vi "Stepper motor-Example.vi"() -> ()   [LabVIEW 2013]
uses:
  <vilib>/LabVIEW Interface for Arduino/Type Defs/Connection Type.ctl
  <vilib>/LabVIEW Interface for Arduino/Type Defs/Board Type.ctl
  <vilib>/LabVIEW Interface for Arduino/LabVIEW Interface for Arduino.lvlib
panel:
  in  "?":bool
  in  "RPM Control":dbl(knob) scale=0.0..6.0
  in  "Continuious Mode":bool
  in  "Half Step":bool
  in  "CW":bool
  # "Control Panel"
  # "CCW"
  # "Full Step"
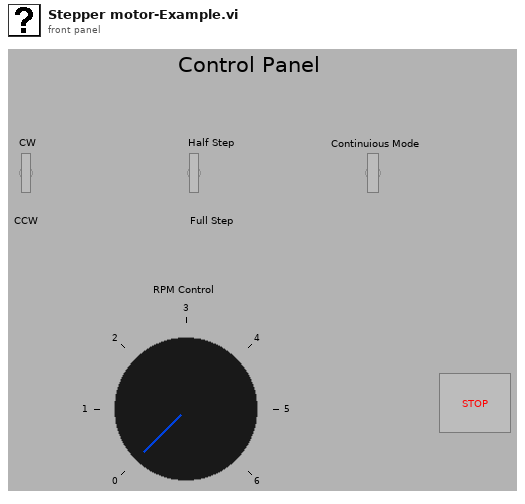
[diagram p1: front panel]
types:
  T1 = typedef "LabVIEW Interface for Arduino.lvlib/Board Type.ctl" = enum16{"Uno", "Dimuelanove w/Atmega 328", "Mega 2560"}
  T2 = typedef "LabVIEW Interface for Arduino.lvlib/Connection Type.ctl" = enum8{"USB / Serial", "XBEE", "BlueSmirf (Bluetooth)"}
  T3 = typedef "LabVIEW Interface for Arduino.lvlib/Arduino Resource.ctl" = cluster{"VISA resource":refnum<visa-resource-name>, "Board Type":T1, "Connection Type":enum8{"USB / Serial"}, "Bytes Per Packet (15)":u8}
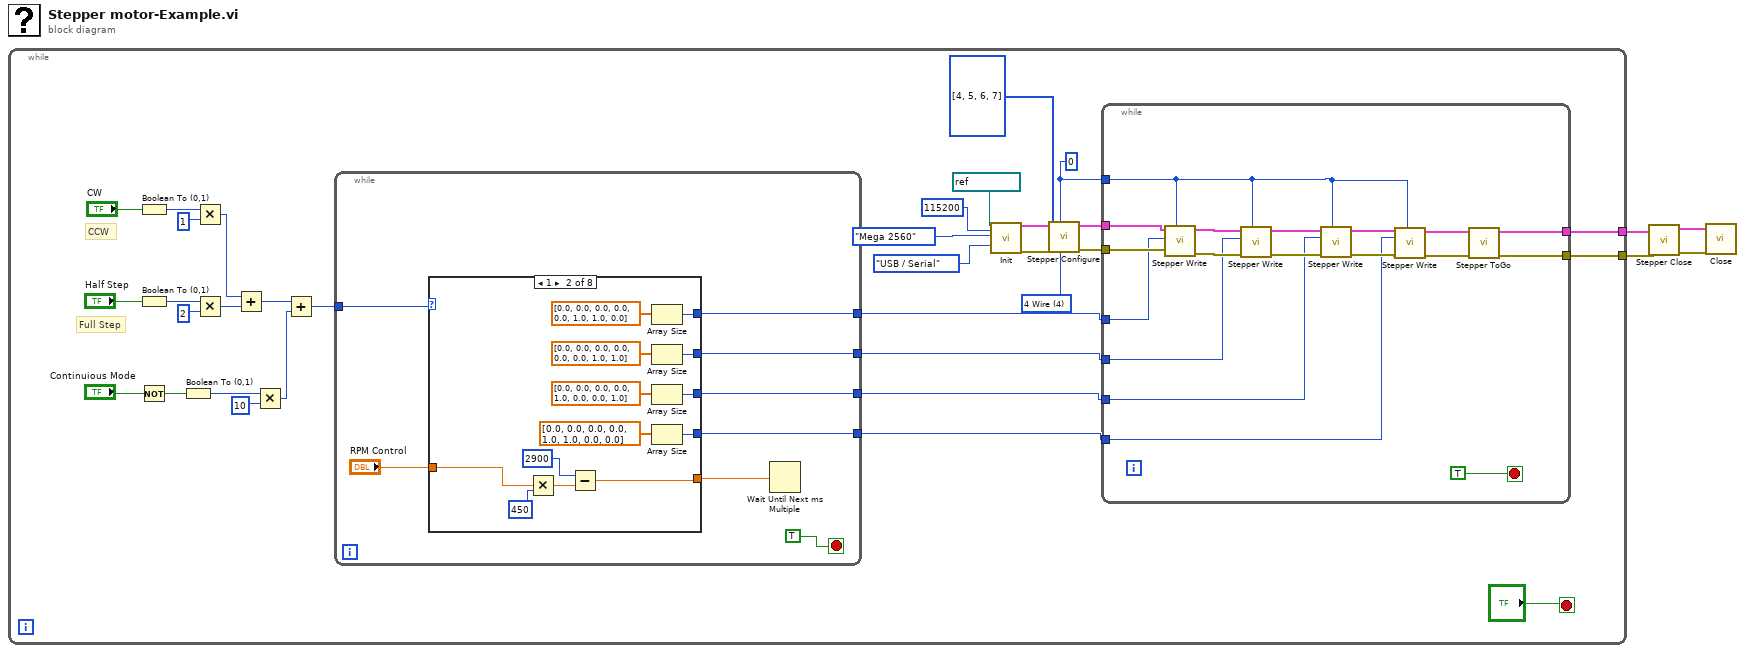
[diagram p0: block diagram]
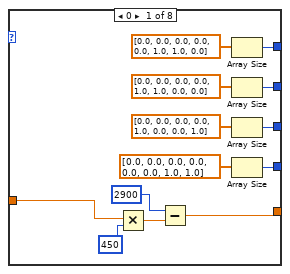
[diagram p2: hidden frame]
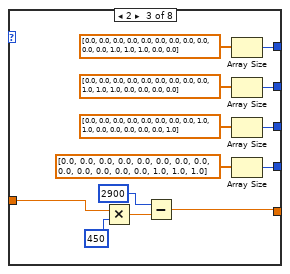
[diagram p3: hidden frame]
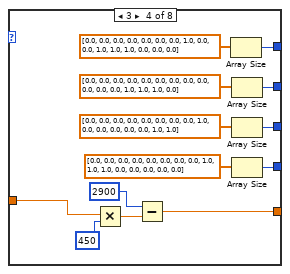
[diagram p4: hidden frame]
diagram:
  n1 = while {
    tunnel: [w6] -> w4
    tunnel: [w5] -> w3
    stop <- "?" stop-if-true
    w17 = u8 4 items=["2 Wire (Pulse & Direction)"=1, "2 Wire"=2, "4 Wire"=4, "EasyDriver"=6, "AF Motor Shield (Stepper 1 & 2 Only)"=5] ("Control Method")
    w21 = u8 0 ("Stepper #")
    # "Full Step"
    # "CCW"
    n2 = Boolean To (0,1)(Boolean="CW") -> (0, 1=w37:i16)
    n3 = Boolean To (0,1)(Boolean="Half Step") -> (0, 1=w34:i16)
    n4 = Not(x="Continuious Mode") -> (.not. x?=w31:bool)
    n5 = Boolean To (0,1)(Boolean=w31) -> (0, 1=w29:i16)
    n6 = Multiply(x=w37, y=1) -> (x*y=w30:i32)
    n7 = Multiply(x=w34, y=2) -> (x*y=w25:i32)
    n8 = Add(x=w30, y=w25) -> (x+y=w27:i32)
    n9 = Multiply(x=w29, y=10) -> (x*y=w26:i32)
    n10 = Add(x=w27, y=w26) -> (x+y=w23:i32)
    n11 = while {
      tunnel: w23 -> [w61]
      tunnel: [w59] -> w11
      tunnel: [w58] -> w10
      tunnel: [w57] -> w9
      tunnel: [w56] -> w8
      stop <- TRUE stop-if-true
      n12 = case "CW Full" shown="1" w61 {
        tunnel: [w72 w85 w98 w111 _ _ _ _] -> w56
        tunnel: [w71 w84 w97 w110 _ _ _ _] -> w58
        tunnel: [w70 w83 w96 w109 _ _ _ _] -> w57
        tunnel: [w69 w82 w95 w108 _ _ _ _] -> w59
        tunnel: "RPM Control" -> [w65 w78 w91 w103 _ _ _ _]
        tunnel: [w64 w77 w90 w106 _ _ _ _] -> w62
        frame 0 {
          n13 = Multiply(x=w65, y=450) -> (x*y=w67:dbl)
          n14 = Subtract(x=2900, y=w67) -> (x-y=w64:dbl)
          n15 = Array Size(array=dbl[] [0.0, 0.0, 0.0, 0.0, 0.0, 1.0, 1.0, 0.0]) -> (size(s)=w69:i32)
          n16 = Array Size(array=dbl[] [0.0, 0.0, 0.0, 0.0, 1.0, 1.0, 0.0, 0.0]) -> (size(s)=w71:i32)
          n17 = Array Size(array=dbl[] [0.0, 0.0, 0.0, 0.0, 1.0, 0.0, 0.0, 1.0]) -> (size(s)=w70:i32)
          n18 = Array Size(array=dbl[] [0.0, 0.0, 0.0, 0.0, 0.0, 0.0, 1.0, 1.0]) -> (size(s)=w72:i32)
        }
        frame 1 {
          n19 = Multiply(x=w78, y=450) -> (x*y=w80:dbl)
          n20 = Subtract(x=2900, y=w80) -> (x-y=w77:dbl)
          n21 = Array Size(array=dbl[] [0.0, 0.0, 0.0, 0.0, 0.0, 1.0, 1.0, 0.0]) -> (size(s)=w82:i32)
          n22 = Array Size(array=dbl[] [0.0, 0.0, 0.0, 0.0, 0.0, 0.0, 1.0, 1.0]) -> (size(s)=w84:i32)
          n23 = Array Size(array=dbl[] [0.0, 0.0, 0.0, 0.0, 1.0, 0.0, 0.0, 1.0]) -> (size(s)=w83:i32)
          n24 = Array Size(array=dbl[] [0.0, 0.0, 0.0, 0.0, 1.0, 1.0, 0.0, 0.0]) -> (size(s)=w85:i32)
        }
        frame 2 {
          n25 = Multiply(x=w91, y=450) -> (x*y=w93:dbl)
          n26 = Subtract(x=2900, y=w93) -> (x-y=w90:dbl)
          n27 = Array Size(array=dbl[] [0.0, 0.0, 0.0, 0.0, 0.0, 0.0, 0.0, 0.0, 0.0, 0.0, 0.0, 1.0, 1.0, 1.0, 0.0, 0.0]) -> (size(s)=w95:i32)
          n28 = Array Size(array=dbl[] [0.0, 0.0, 0.0, 0.0, 0.0, 0.0, 0.0, 0.0, 0.0, 1.0, 1.0, 1.0, 0.0, 0.0, 0.0, 0.0]) -> (size(s)=w97:i32)
          n29 = Array Size(array=dbl[] [0.0, 0.0, 0.0, 0.0, 0.0, 0.0, 0.0, 0.0, 1.0, 1.0, 0.0, 0.0, 0.0, 0.0, 0.0, 1.0]) -> (size(s)=w96:i32)
          n30 = Array Size(array=dbl[] [0.0, 0.0, 0.0, 0.0, 0.0, 0.0, 0.0, 0.0, 0.0, 0.0, 0.0, 0.0, 0.0, 1.0, 1.0, 1.0]) -> (size(s)=w98:i32)
        }
        frame 3 {
          n31 = Multiply(x=w103, y=450) -> (x*y=w105:dbl)
          n32 = Subtract(x=2900, y=w105) -> (x-y=w106:dbl)
          n33 = Array Size(array=dbl[] [0.0, 0.0, 0.0, 0.0, 0.0, 0.0, 0.0, 1.0, 0.0, 0.0, 1.0, 1.0, 1.0, 0.0, 0.0, 0.0]) -> (size(s)=w108:i32)
          n34 = Array Size(array=dbl[] [0.0, 0.0, 0.0, 0.0, 0.0, 0.0, 0.0, 0.0, 0.0, 0.0, 0.0, 0.0, 1.0, 1.0, 1.0, 0.0]) -> (size(s)=w110:i32)
          n35 = Array Size(array=dbl[] [0.0, 0.0, 0.0, 0.0, 0.0, 0.0, 0.0, 0.0, 1.0, 0.0, 0.0, 0.0, 0.0, 0.0, 1.0, 1.0]) -> (size(s)=w109:i32)
          n36 = Array Size(array=dbl[] [0.0, 0.0, 0.0, 0.0, 0.0, 0.0, 0.0, 0.0, 1.0, 1.0, 1.0, 0.0, 0.0, 0.0, 0.0, 0.0]) -> (size(s)=w111:i32)
        }
        frame 10 {
        }
        frame 11 {
        }
        frame 12 {
        }
        frame 13, Default {
        }
      }
      n37 = Wait Until Next ms Multiple(millisecond multiple=w62) -> ()  [unwired: 1 out]
    }
    n38 = call <vilib>:"Init.vi"("VISA resource"=refnum<visa-resource-name> "COM10", "Baud Rate (115200)"=u32 115200, "Board Type (Uno)"=Board_Type."Mega 2560", "Connection Type (USB/Serial)"=Connection_Type."USB / Serial") -> ("Arduino Resource"=w15:T3, "error out"=w16:errorcluster)  [unwired: 14 in]
    n39 = call <vilib>:"Stepper Configure.vi"("Control Method"=w17, "Stepper #"=w21, "error in"=w16, "Stepper Pins"=u8[] [4, 5, 6, 7], "Arduino Resource"=w15) -> ("error out"=w20:errorcluster, "Arduino Resource Out"=w19:T3)  [unwired: 5 in]
    n40 = while {
      tunnel: w19 -> [w55]
      tunnel: w20 -> [w54]
      tunnel: w21 -> [w49]
      tunnel: [w44] -> w6
      tunnel: [w43] -> w5
      tunnel: w11 -> [w42]
      tunnel: w10 -> [w41]
      tunnel: w9 -> [w40]
      tunnel: w8 -> [w39]
      stop <- TRUE stop-if-true
      n41 = call <vilib>:"Stepper Write.vi"("Stepper #"=w49, "error in"=w54, "# of Steps to Move"=w42, "Arduino Resource"=w55) -> ("error out"=w53:errorcluster, "Arduino Resource Out"=w52:T3)  [unwired: 6 in]
      n42 = call <vilib>:"Stepper Write.vi"("Stepper #"=w49, "error in"=w53, "# of Steps to Move"=w41, "Arduino Resource"=w52) -> ("error out"=w51:errorcluster, "Arduino Resource Out"=w50:T3)  [unwired: 6 in]
      n43 = call <vilib>:"Stepper Write.vi"("Stepper #"=w49, "error in"=w51, "# of Steps to Move"=w40, "Arduino Resource"=w50) -> ("error out"=w47:errorcluster, "Arduino Resource Out"=w48:T3)  [unwired: 6 in]
      n44 = call <vilib>:"Stepper Write.vi"("Stepper #"=w49, "error in"=w47, "# of Steps to Move"=w39, "Arduino Resource"=w48) -> ("error out"=w45:errorcluster, "Arduino Resource Out"=w46:T3)  [unwired: 6 in]
      n45 = call <vilib>:"Stepper ToGo.vi"("error in"=w45, "Arduino Resource"=w46) -> ("error out"=w43:errorcluster, "Arduino Resource Out"=w44:T3)  [unwired: 6 in, 2 out]
    }
  }
  n46 = call <vilib>:"Stepper Close.vi"("error in"=w3, "Arduino Resource"=w4) -> ("error out"=w2:errorcluster, "Arduino Resource Out"=w1:T3)  [unwired: 8 in]
  n47 = call <vilib>:"Close.vi"("Arduino Resource"=w1, "error in"=w2) -> ()  [unwired: 13 in, 1 out]
